vi "Rendezvous.vi"() -> ()   [LabVIEW 2011]
panel:
  in  "stop":bool
  out "Task 2#":dbl(graph)
  out "Task 1#":dbl(graph)
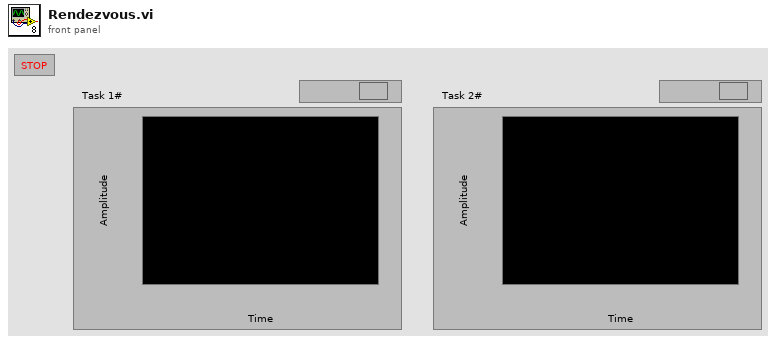
[diagram p1: front panel]
types:
  T1 = typedef "Rendezvous RefNum" = refnum<k1>
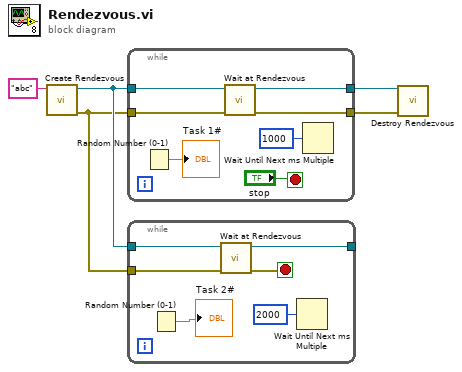
[diagram p0: block diagram]
diagram:
  n1 = call <vilib>:"Create Rendezvous.vi"("name (unnamed)"="abc") -> ("error out"=w1:errorcluster, "rendezvous"=w2:T1)  [unwired: 4 in, 1 out]
  n2 = while {
    tunnel: w2 -> [w11]
    tunnel: w1 -> [w10]
    tunnel: [w9] -> w5
    tunnel: [w8] -> w4
    stop <- "stop" stop-if-true
    n3 = Random Number (0-1)() -> (number: 0 to 1=→"Task 1#":dbl)
    n4 = call <vilib>:"Wait at Rendezvous.vi"("error in (no error)"=w10, "rendezvous"=w11) -> ("error out"=w8:errorcluster, "rendezvous out"=w9:T1)  [unwired: 3 in, 1 out]
    n5 = Wait Until Next ms Multiple(millisecond multiple=u32 1000) -> ()  [unwired: 1 out]
  }
  n6 = while {
    tunnel: w2 -> [w18]
    tunnel: w1 -> [w17]
    tunnel: [w15] -> _
    stop <- w14 stop-if-true
    n7 = Random Number (0-1)() -> (number: 0 to 1=→"Task 2#":dbl)
    n8 = call <vilib>:"Wait at Rendezvous.vi"("error in (no error)"=w17, "rendezvous"=w18) -> ("error out"=w14:errorcluster, "rendezvous out"=w15:T1)  [unwired: 3 in, 1 out]
    n9 = Wait Until Next ms Multiple(millisecond multiple=u32 2000) -> ()  [unwired: 1 out]
  }
  n10 = call <vilib>:"Destroy Rendezvous.vi"("error in (no error)"=w4, "rendezvous"=w5) -> ()  [unwired: 4 in, 2 out]
